vi "VCM_Merge_Cluster.vi"(1 "VCM Control":T2, 2 "VCM Status":T1) -> (0 "VCM Monitor":T3)   [LabVIEW 2019]
uses:
  Mischer/VCM-Cluster.ctl
  Mischer/VCM-Control.ctl
  Mischer/VCM-Status.ctl
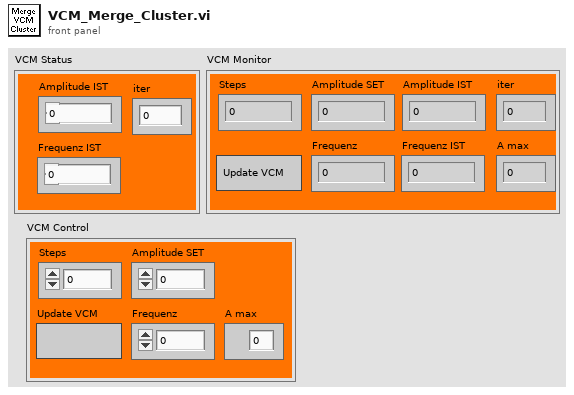
[diagram p1: front panel]
types:
  T1 = typedef "VCM-Status.ctl" = cluster{"Amplitude IST":dbl, "Frequenz IST":dbl, "iter":dbl}
  T2 = typedef "VCM-Control.ctl" = cluster{"Steps":dbl, "Amplitude SET":dbl, "Frequenz":dbl, "A max":dbl, "Update VCM":bool}
  T3 = typedef "VCM-Cluster.ctl" = cluster{"Steps":dbl, "Amplitude SET":dbl, "Frequenz":dbl, "Amplitude IST":dbl, "Frequenz IST":dbl, "A max":dbl, "iter":dbl, "Update VCM":bool}
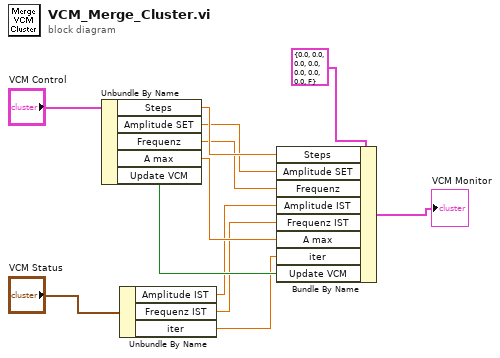
[diagram p0: block diagram]
diagram:
  n1 = Unbundle By Name("VCM Control") -> ("Steps"=w8:dbl, "Amplitude SET"=w7:dbl, "Frequenz"=w6:dbl, "A max"=w5:dbl, "Update VCM"=w4:bool)
  n2 = Unbundle By Name("VCM Status") -> ("Amplitude IST"=w3:dbl, "Frequenz IST"=w2:dbl, "iter"=w1:dbl)
  n3 = Bundle By Name(cluster=T3 {"Steps"=0.0, "Amplitude SET"=0.0, "Frequenz"=0.0, "Amplitude IST"=0.0, "Frequenz IST"=0.0, "A max"=0.0, "iter"=0.0, "Update VCM"=FALSE} ("VCM Monitor 2"), "Steps"=w8, "Amplitude SET"=w7, "Frequenz"=w6, "Amplitude IST"=w3, "Frequenz IST"=w2, "A max"=w5, "iter"=w1, "Update VCM"=w4) -> (→"VCM Monitor":T3)
